vi "AnotherInsertExample.vi"   [LabVIEW 2017]
uses:
  <vilib>/addons/database/Connection.llb/DB Tools Open Connec (Path).vi
  <vilib>/addons/database/NI_Database_API.lvlib
types:
  T1 = typedef "NI_Database_API.lvlib/Conn ObjectReference.ctl" = refnum<k1>
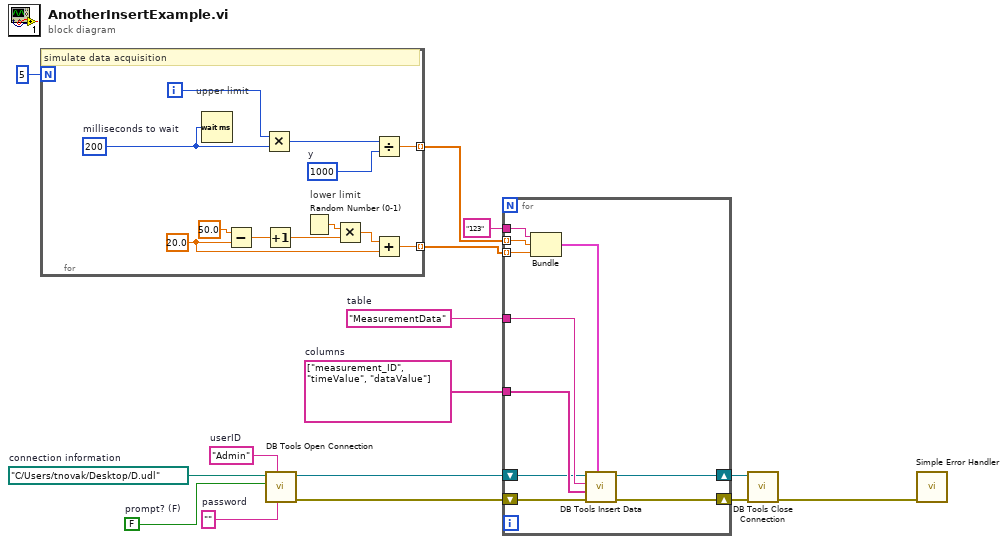
[diagram p0: block diagram]
diagram:
  w10 = string[] ["measurement_ID", "timeValue", "dataValue"]  # columns
  w11 = "MeasurementData"  # table
  w15 = path "C:/Users/tnovak/Desktop/D.udl"  # connection information
  w12 = ""  # password
  w14 = FALSE  # prompt? (F)
  w13 = "Admin"  # userID
  n1 = for {
    N: 5 -> [_]
    tunnel: [w21] -> w2 mode=indexing
    tunnel: [w16] -> w3 mode=indexing
    i -> [w20]
    w17 = u32 1000  # y
    w22 = 20.0
    w19 = u32 200  # milliseconds to wait
    # "lower limit"
    # "upper limit"
    # "simulate data acquisition"
    n2 = Wait (ms)(milliseconds to wait=w19) -> ()  [unwired: 1 out]
    n3 = Subtract(x=50.0, y=w22) -> (x-y=w25:dbl)
    n4 = Multiply(x=w20, y=w19) -> (x*y=w18:u32)
    n5 = Increment(x=w25) -> (x+1=w24:dbl)
    n6 = Random Number (0-1)() -> (number: 0 to 1=w27:dbl)
    n7 = Multiply(x=w27, y=w24) -> (x*y=w23:dbl)
    n8 = Divide(x=w18, y=w17) -> (x/y=w16:dbl)
    n9 = Add(x=w23, y=w22) -> (x+y=w21:dbl)
  }
  n10 = call-poly <vilib>:"DB Tools Open Connection.vi"("password"=w12, "userID"=w13, "prompt? (F)"=w14, "connection information"=w15) -> ("error out"=w7:errorcluster, "connection reference"=w8:T1)  [unwired: 4 in]
  n11 = for {
    tunnel: w11 -> [w37]
    tunnel: w10 -> [w36]
    shift-right: [w32] -> w5
    shift-left: w8 -> [w35]
    shift-right: [w33] -> w6
    shift-left: w7 -> [w34]
    tunnel: w3 -> [w31] mode=indexing
    tunnel: w2 -> [w30] mode=indexing
    tunnel: "123" -> [w29]
    n12 = Bundle(w29, w31, w30) -> (w28:cluster{string, dbl, dbl})  [unwired: 1 in]
    n13 = call <vilib>:"DB Tools Insert Data.vi"("data"=w28, "error in (no error)"=w34, "columns"=w36, "table"=w37, "connection reference"=w35) -> ("error out"=w33:errorcluster, "connection reference out"=w32:T1)  [unwired: 5 in]
  }
  n14 = call <vilib>:"DB Tools Close Connection.vi"("error in (no error)"=w6, "connection reference"=w5) -> ("error out"=w9:errorcluster)  [unwired: 5 in]
  n15 = call <vilib>:"Simple Error Handler.vi"("error in (no error)"=w9) -> ()  [unwired: 4 in, 5 out]
